vi "2023 Increment teleopCounter.vi"(1 "error in":errorcluster) -> (0 "error out":errorcluster)   [LabVIEW 2020]
uses:
  2023 Robot Global Data.vi
panel:
  out "teleopCounter":i32
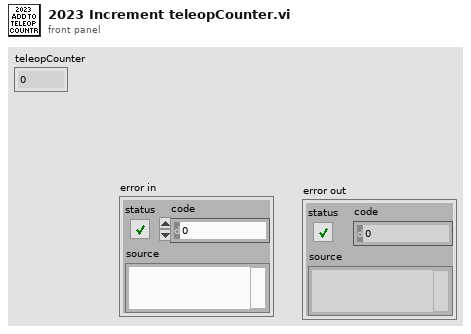
[diagram p1: front panel]
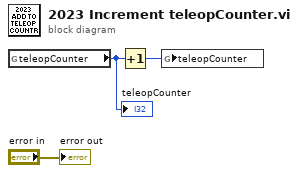
[diagram p0: block diagram]
diagram:
  n1 = global read "2023 Robot Global Data.vi" "teleopCounter"() -> (w3:i32)
  "teleopCounter" <- w3
  n2 = Increment(x=w3) -> (x+1=w2:i32)
  n3 = global write "2023 Robot Global Data.vi" "teleopCounter"(w2) -> ()
  "error out" <- "error in"
